vi "בדיקת מפל מתח בין הדקי הממסר תחת עומס 4.vi"(8 "error":errorcluster, 11 "Path for Log":path) -> (0 "error IO":errorcluster, 1 "בטווח כן/לא":bool, 2 "מפל מתח בין דקי הממסר תחת עומס":dbl, 3 "תוצאה זמנית":dbl)   [LabVIEW 2014]
uses:
  M9700 Driver/85/vi.lib/M9700 Modbus.llb/CTL Register Address.ctl
  M9700 Driver/86/vi.lib/M9700 Modbus.llb/CTL CMD Register.ctl
  <vilib>/DAQmx/create/channels.llb/DAQmx Create Channel (DO-Digital Output).vi
  <vilib>/DAQmx/write.llb/DAQmx Write (Digital Bool 1Line 1Point).vi
panel:
  out "progress":dbl(slide) min=0.0 max=10.0 scale=0.0..10.0
  in  "stop":bool
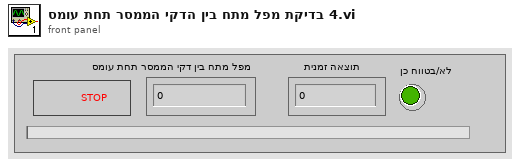
[diagram p1: front panel]
types:
  T1 = enum32{"Invalid", "Standard", "Closed", "Hidden", "Minimized", "Maximized"}
  T2 = typedef "CTL CMD Register.ctl" = u8
  T3 = typedef "CTL Register Address.ctl" = u16
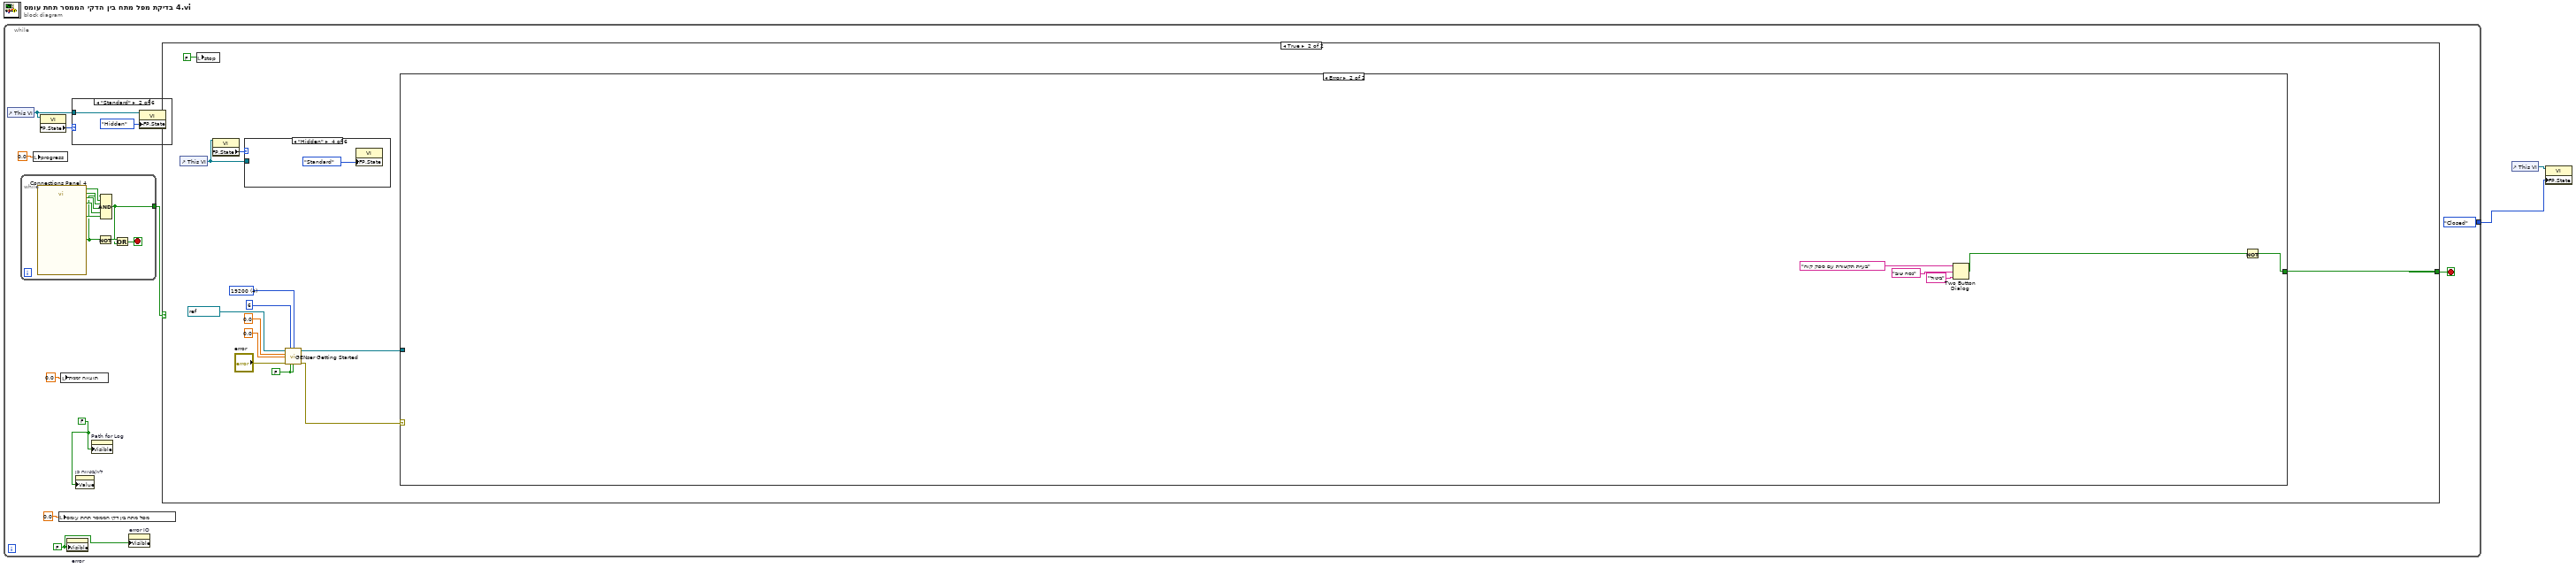
[diagram p0: block diagram]
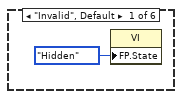
[diagram p2: hidden frame]
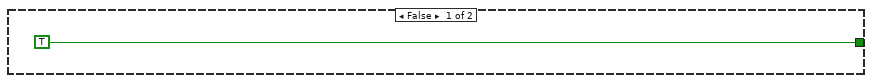
[diagram p7: hidden frame]
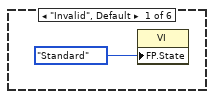
[diagram p8: hidden frame]
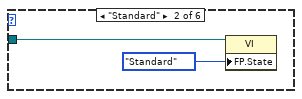
[diagram p9: hidden frame]
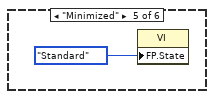
[diagram p11: hidden frame]
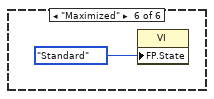
[diagram p12: hidden frame]
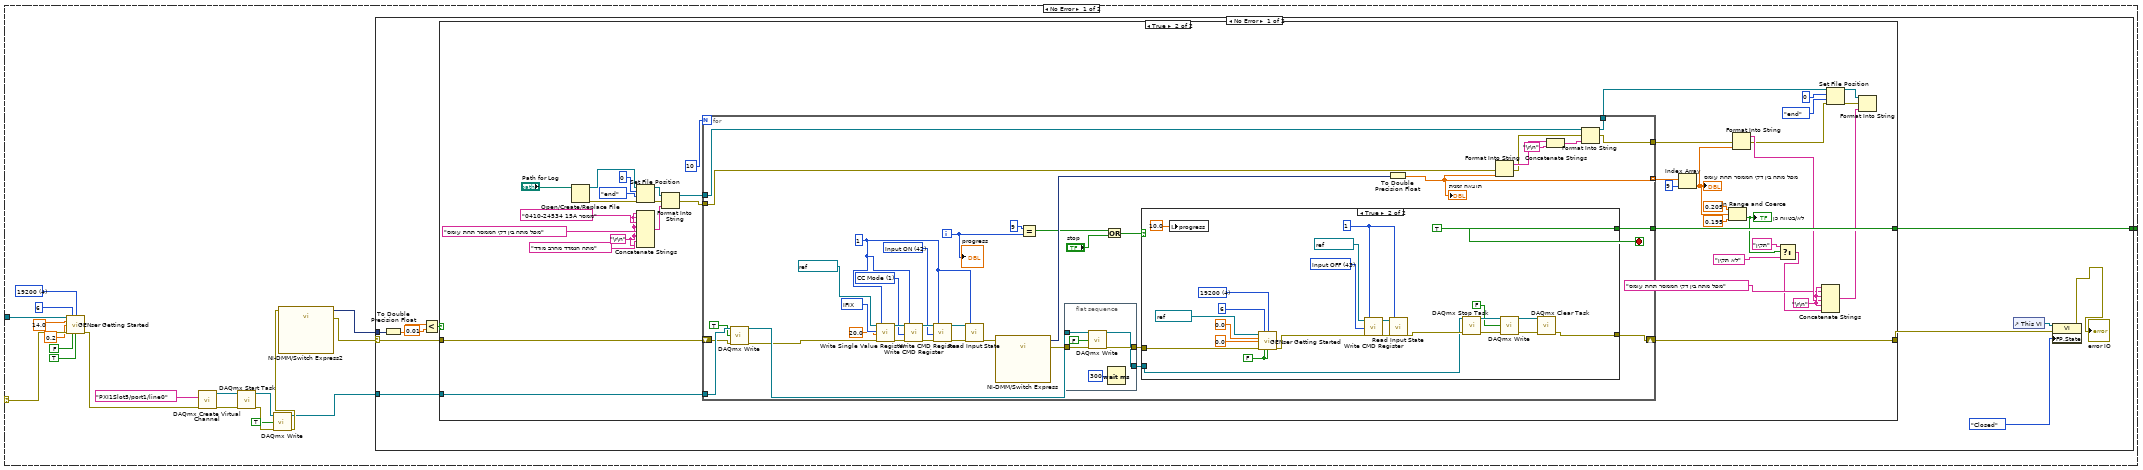
[diagram p13: hidden frame]
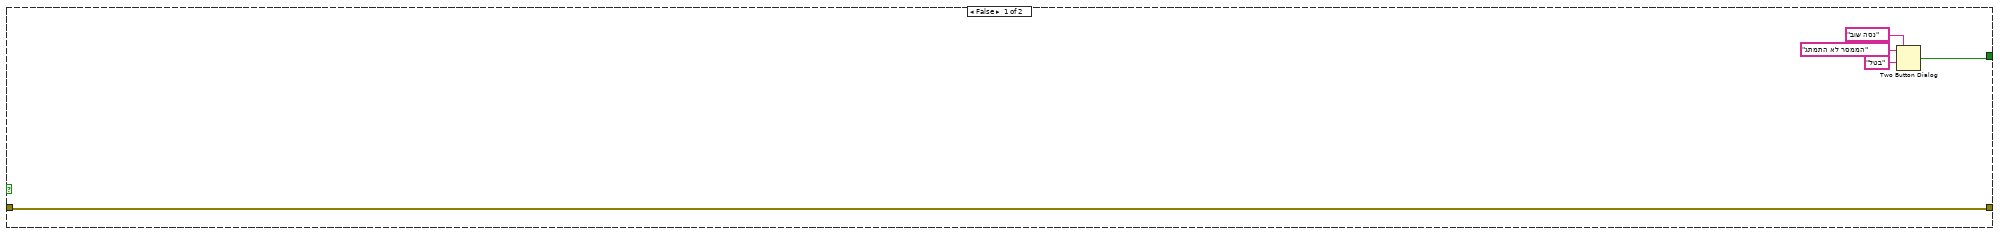
[diagram p14: hidden frame]
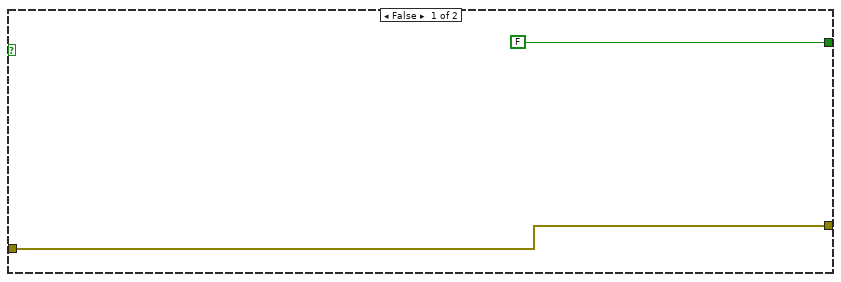
[diagram p15: hidden frame]
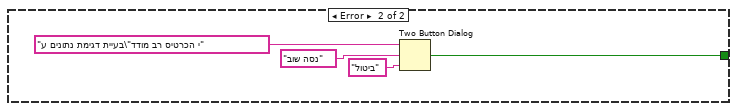
[diagram p16: hidden frame]
diagram:
  n1 = while {
    tunnel: [T1."Closed" ("Front Panel Window:State")] -> w1
    stop <- w4 stop-if-true
    w5 = FALSE ("Visible")
    w8 = FALSE ("Visible")
    n2 = control-ref of="This VI"() -> (w7:refnum<vi>)
    n3 = while {
      tunnel: [w13] -> w12
      stop <- w16 stop-if-true
      n4 = call "Connections Panel 4.vi"() -> ("Input Name 10"=w17:bool, "Input Name 6"=w21:bool, "Input Name 7"=w20:bool, "Input Name 8"=w19:bool, "Input Name 9"=w18:bool, "OK"=w14:bool)  [unwired: 13 in, 1 out]
      n5 = Not(x=w14) -> (.not. x?=w15:bool)
      n6 = Compound Arithmetic op=AND(w14, w21, w20, w19, w18, w17) -> (w13:bool)
      n7 = Or(x=w15, y=w13) -> (x .or. y?=w16:bool)
    }
    n8 = local write "progress"(0.0 ("progress")) -> ()
    n9 = property class="VI"(reference=w7) -> ("FP.State"=w6:T1)  [unwired: 1 in, 2 out]
    n10 = local write "מפל מתח בין דקי הממסר תחת עומס"(0.0 ("מפל מתח בין דקי הממסר תחת עומס")) -> ()
    n11 = local write "תוצאה זמנית"(0.0 ("תוצאה זמנית")) -> ()
    n12 = property on="error" class="Clust (strict)"("Visible"=w8) -> ()  [unwired: 2 in, 2 out]
    n13 = case shown="\"Standard\"" w6 {
      tunnel: w7 -> [_ w23 _ _ _ _]
      frame "Invalid", Default {
        n14 = property class="VI"("FP.State"=T1."Hidden" ("Front Panel Window:State")) -> ()  [unwired: 2 in, 2 out]
      }
      frame "Standard" {
        n15 = property class="VI"(reference=w23, "FP.State"=T1."Hidden" ("Front Panel Window:State")) -> ()  [unwired: 1 in, 2 out]
      }
      frame "Closed" {
      }
      frame "Hidden" {
      }
      frame "Minimized" {
      }
      frame "Maximized" {
      }
    }
    n16 = property on="בטווח כן/לא" class="Bool (strict)"("Value"=w5) -> ()  [unwired: 2 in, 2 out]
    n17 = property on="Path for Log" class="Path"("Visible"=w5) -> ()  [unwired: 2 in, 2 out]
    n18 = property on="error IO" class="Clust (strict)"("Visible"=w8) -> ()  [unwired: 2 in, 2 out]
    n19 = case shown="True" w12 {
      tunnel: [TRUE w26] -> w4
      frame False {
      }
      frame True {
        w31 = FALSE ("Output On (T)")
        w35 = u16 4 items=["1200", "2400", "4800", "9600", "19200"] ("BAUD")
        n20 = control-ref of="This VI"() -> (w28:refnum<vi>)
        n21 = local write "stop"(FALSE ("stop")) -> ()
        n22 = property class="VI"(reference=w28) -> ("FP.State"=w29:T1)  [unwired: 1 in, 2 out]
        n23 = case shown="\"Hidden\"" w29 {
          tunnel: w28 -> [_ w40 _ _ _ _]
          frame "Invalid", Default {
            n24 = property class="VI"("FP.State"=T1."Standard" ("Front Panel Window:State")) -> ()  [unwired: 2 in, 2 out]
          }
          frame "Standard" {
            n25 = property class="VI"(reference=w40, "FP.State"=T1."Standard" ("Front Panel Window:State")) -> ()  [unwired: 1 in, 2 out]
          }
          frame "Closed" {
          }
          frame "Hidden" {
            n26 = property class="VI"("FP.State"=T1."Standard" ("Front Panel Window:State")) -> ()  [unwired: 2 in, 2 out]
          }
          frame "Minimized" {
            n27 = property class="VI"("FP.State"=T1."Standard" ("Front Panel Window:State")) -> ()  [unwired: 2 in, 2 out]
          }
          frame "Maximized" {
            n28 = property class="VI"("FP.State"=T1."Standard" ("Front Panel Window:State")) -> ()  [unwired: 2 in, 2 out]
          }
        }
        n29 = call "GENser Getting Started.vi"("VISA"=refnum<visa-resource-name> "COM6", "GEN Addr"=i16 6, "BAUD"=w35, "Voltage Limit"=0.0, "Current Limit"=0.0, "error"="error", "Reset (T)"=w31, "Output On (T)"=w31) -> ("VISA out"=w37:refnum<visa-resource-name>, "error out"=w27:errorcluster)  [unwired: 4 in, 2 out]
        n30 = case shown="Error" w27 {
          selector: w27 -> [w61 _]
          tunnel: w37 -> [w64 _]
          tunnel: [w63 w193] -> w26
          frame No Error {
            w55 = u16 4 items=["1200", "2400", "4800", "9600", "19200"] ("BAUD")
            n31 = call "GENser Getting Started.vi"("VISA"=w64, "GEN Addr"=i16 6, "BAUD"=w55, "Voltage Limit"=14.0, "Current Limit"=0.2, "error"=w61, "Reset (T)"=FALSE, "Output On (T)"=TRUE) -> ("error out"=w47:errorcluster)  [unwired: 4 in, 3 out]
            n32 = call-poly <vilib>:"DAQmx Create Virtual Channel.vi"("lines"=tag "PXI1Slot5/port1/line0", "error in"=w47) -> ("task out"=w53:refnum<k21>, "error out"=w54:errorcluster)  [unwired: 12 in]
            n33 = call <vilib>:"DAQmx Start Task.vi"("task/channels in"=w53, "error in"=w54) -> ("task out"=w46:refnum<k21>, "error out"=w49:errorcluster)  [unwired: 12 in]
            n34 = call-poly <vilib>:"DAQmx Write.vi"("task/channels in"=w46, "data"=TRUE, "error in"=w49) -> ("task out"=w45:refnum<k21>, "error out"=w50:errorcluster)  [unwired: 10 in, 1 out]
            n35 = call "NI-DMM/Switch Express2"("error in"=w50) -> ("signals out"=w62:dynamicdata, "error out"=w51:errorcluster)  [unwired: 16 in, 1 out]
            n36 = case shown="No Error" w51 {
              selector: w51 -> [w73 _]
              tunnel: [w72 w189] -> w63
              tunnel: w62 -> [w75 _]
              tunnel: w45 -> [w66 _]
              frame No Error {
                n37 = To Double Precision Float(number=w75) -> (double precision float=w71:dbl)
                n38 = Less?(x=w71, y=0.01) -> (x < y?=w74:bool)
                n39 = case shown="True" w74 {
                  tunnel: w73 -> [w80 w117]
                  tunnel: [w79 w118] -> w72
                  tunnel: [w80 w111] -> w67
                  tunnel: w66 -> [_ w112]
                  frame False {
                    n40 = Two Button Dialog(message="הממסר לא התמתג", 1:"נסה שוב" ("F button name (\"Cancel\")"), 2:"בטל" ("T button name (\"OK\")")) -> (T button?=w79:bool)
                  }
                  frame True {
                    w96 = "\r\n"
                    w99 = "\r\n"
                    n41 = Open/Create/Replace File(file path (use dialog)="Path for Log") -> (refnum out=w108:refnum<file>, error out=w107:errorcluster)  [unwired: 5 in, 1 out]
                    n42 = Set File Position(offset (in bytes) (0)=i64 0, refnum=w108, from (0:start)=enum16{"start", "end", "current"}."end", error in=w107) -> (refnum out=w103:refnum<file>, error out=w100:errorcluster)
                    n43 = Concatenate Strings(w99, w99, "0410-24534 15A ממסר", w99, "מפל מתח בין דקי הממסר תחת עומס", w99, "מתח הנמדד מהרב מודד", w99) -> (w106:string)
                    n44 = Format Into String(initial string=w103, error in=w100, w106) -> (resulting string=w97:refnum<file>, error out=w98:errorcluster)  [unwired: 1 in]
                    n45 = for {
                      N: 10 -> [_]
                      tunnel: [w140] -> w118
                      shift-right: [w138] -> w111
                      shift-left: w117 -> [w133]
                      tunnel: [w121] -> w116 mode=indexing
                      tunnel: w112 -> [w134]
                      tunnel: w98 -> [w124]
                      tunnel: w97 -> [w126]
                      tunnel: [w123] -> w90
                      tunnel: [w122] -> w81
                      i -> [w137]
                      stop <- w140 stop-if-true
                      w148 = T2 42 items=["CC Mode"=1, "CV Mode"=2, "CW Mode"=3, "CR Mode"=4, "Short Mode"=26, "Set SysPara"=41, "Input ON"=42, "Input OFF"=43] ("CMD Register Value")
                      w151 = u8 1 ("Load Address")
                      w154 = T2 1 items=["CC Mode"=1, "CV Mode"=2, "CW Mode"=3, "CR Mode"=4, "Short Mode"=26, "Set SysPara"=41, "Input ON"=42, "Input OFF"=43] ("CMD Register Value")
                      w157 = T3 2561 items=["REMOTE"=1283, "ISTATE"=1296, "CMD"=2560, "IFIX"=2561, "UFIX"=2563, "PFIX"=2565, "RFIX"=2567, "IMAX"=2612, "UMAX"=2614, "PMAX"=2616, "U"=2816, "I"=2818, "MODEL"=2822, "EDITION"=2823] ("Register Address")
                      n46 = call-poly <vilib>:"DAQmx Write.vi"("task/channels in"=w134, "data"=TRUE, "error in"=w133) -> ("task out"=w132:refnum<k21>, "error out"=w120:errorcluster)  [unwired: 10 in, 1 out]
                      n47 = call "Write Single Value Register.vi"("VISA resource name"=refnum<visa-resource-name> "COM13", "Starting Address(HEX)"=w157, "Register Single Value"=sgl 20.0, "error in"=w120, "Load Address"=w151) -> ("VISA resource name out"=w156:refnum<visa-resource-name>, "error out"=w155:errorcluster)  [unwired: 13 out]
                      n48 = call "Write CMD Register.vi"("VISA resource name"=w156, "CMD Value"=w154, "error in"=w155, "Load Address"=w151) -> ("VISA resource name out"=w152:refnum<visa-resource-name>, "error out"=w149:errorcluster)  [unwired: 14 out]
                      n49 = call "Write CMD Register.vi"("VISA resource name"=w152, "CMD Value"=w148, "error in"=w149, "Load Address"=w151) -> ("VISA resource name out"=w150:refnum<visa-resource-name>, "error out"=w147:errorcluster)  [unwired: 14 out]
                      n50 = call "Read Input State.vi"("VISA resource name"=w150, "error in"=w147, "Load Address"=w151) -> ("error out"=w146:errorcluster)  [unwired: 16 out]
                      n51 = call "NI-DMM/Switch Express"("error in"=w146) -> ("signals out"=w145:dynamicdata, "error out"=w135:errorcluster)  [unwired: 16 in, 1 out]
                      n52 = Equal?(x=9, y=w137) -> (x = y?=w142:bool)
                      n53 = flat-sequence {
                        tunnel: [w163] -> w136
                        tunnel: w135 -> [w162]
                        tunnel: w132 -> [w160]
                        tunnel: [w159] -> w130
                        frame #0 {
                          n54 = call-poly <vilib>:"DAQmx Write.vi"("task/channels in"=w160, "data"=FALSE, "error in"=w162) -> ("task out"=w159:refnum<k21>, "error out"=w163:errorcluster)  [unwired: 10 in, 1 out]
                          n55 = Wait (ms)(milliseconds to wait=u32 300) -> ()  [unwired: 1 out]
                        }
                      }
                      n56 = Or(x=w142, y="stop") -> (x .or. y?=w143:bool)
                      n57 = case shown="True" w143 {
                        tunnel: [FALSE TRUE] -> w140
                        tunnel: w136 -> [w164 w182]
                        tunnel: [w164 w168] -> w138
                        tunnel: w130 -> [_ w167]
                        frame False {
                        }
                        frame True {
                          w176 = u8 1 ("Load Address")
                          w179 = T2 43 items=["CC Mode"=1, "CV Mode"=2, "CW Mode"=3, "CR Mode"=4, "Short Mode"=26, "Set SysPara"=41, "Input ON"=42, "Input OFF"=43] ("CMD Register Value")
                          w181 = FALSE ("Reset (T)")
                          w184 = u16 4 items=["1200", "2400", "4800", "9600", "19200"] ("BAUD")
                          n58 = local write "progress"(10.0 ("progress")) -> ()
                          n59 = call "GENser Getting Started.vi"("VISA"=refnum<visa-resource-name> "COM6", "GEN Addr"=i16 6, "BAUD"=w184, "Voltage Limit"=0.0, "Current Limit"=0.0, "error"=w182, "Reset (T)"=w181, "Output On (T)"=w181) -> ("error out"=w166:errorcluster)  [unwired: 4 in, 3 out]
                          n60 = call "Write CMD Register.vi"("VISA resource name"=refnum<visa-resource-name> "COM13", "CMD Value"=w179, "error in"=w166, "Load Address"=w176) -> ("VISA resource name out"=w177:refnum<visa-resource-name>, "error out"=w180:errorcluster)  [unwired: 14 out]
                          n61 = call "Read Input State.vi"("VISA resource name"=w177, "error in"=w180, "Load Address"=w176) -> ("error out"=w169:errorcluster)  [unwired: 16 out]
                          n62 = call <vilib>:"DAQmx Stop Task.vi"("task/channels in"=w167, "error in"=w169) -> ("task out"=w174:refnum<k21>, "error out"=w172:errorcluster)  [unwired: 12 in]
                          n63 = call-poly <vilib>:"DAQmx Write.vi"("task/channels in"=w174, "data"=FALSE, "error in"=w172) -> ("task out"=w171:refnum<k21>, "error out"=w170:errorcluster)  [unwired: 10 in, 1 out]
                          n64 = call <vilib>:"DAQmx Clear Task.vi"("task in"=w171, "error in"=w170) -> ("error out"=w168:errorcluster)  [unwired: 13 in]
                        }
                      }
                      n65 = To Double Precision Float(number=w145) -> (double precision float=w121:dbl)
                      "תוצאה זמנית" <- w121
                      n66 = Format Into String(error in=w124, w121) -> (resulting string=w128:string, error out=w125:errorcluster)  [unwired: 2 in]
                      n67 = Concatenate Strings(w128, "\r\n") -> (w127:string)
                      n68 = Format Into String(initial string=w126, error in=w125, w127) -> (resulting string=w123:refnum<file>, error out=w122:errorcluster)  [unwired: 1 in]
                      "progress" <- w137
                    }
                    n69 = Index Array(array=w116, index=9) -> (element=w89:dbl)
                    "מפל מתח בין דקי הממסר תחת עומס" <- w89
                    n70 = In Range and Coerce(upper limit=0.205, x=w89, lower limit=0.195) -> (In Range?=w84:bool)  [unwired: 1 out]
                    "בטווח כן/לא" <- w84
                    n71 = Format Into String(error in=w81, w89) -> (resulting string=w88:string, error out=w82:errorcluster)  [unwired: 2 in]
                    n72 = Select(t="תקין", s=w84, f="לא תקין") -> (s? t:f=w83:string)
                    n73 = Concatenate Strings(w96, "מפל מתח בין דקי הממסר תחת עומס" ("string"), w96, w88, w96, w83) -> (w91:string)
                    n74 = Set File Position(offset (in bytes) (0)=i64 0, refnum=w90, from (0:start)=enum16{"start", "end", "current"}."end", error in=w82) -> (refnum out=w93:refnum<file>, error out=w92:errorcluster)
                    n75 = Format Into String(initial string=w93, error in=w92, w91) -> ()  [unwired: 1 in, 2 out]
                  }
                }
                n76 = control-ref of="This VI"() -> (w69:refnum<vi>)
                n77 = property class="VI"(reference=w69, error in=w67, "FP.State"=T1."Closed" ("Front Panel Window:State")) -> (error out=→"error IO":errorcluster)  [unwired: 1 out]
              }
              frame Error {
                n78 = Two Button Dialog(message="בעיית דגימת נתונים ע\"י הכרטיס רב מודד", 1:"ביטול" ("F button name (\"Cancel\")"), 2:"נסה שוב" ("T button name (\"OK\")")) -> (T button?=w189:bool)
              }
            }
          }
          frame Error {
            n79 = Two Button Dialog(message="בעיית תקשורת עם ספק קוח", 1:"ביטול" ("F button name (\"Cancel\")"), 2:"נסה שוב" ("T button name (\"OK\")")) -> (T button?=w194:bool)
            n80 = Not(x=w194) -> (.not. x?=w193:bool)
          }
        }
      }
    }
  }
  n81 = control-ref of="This VI"() -> (w2:refnum<vi>)
  n82 = property class="VI"(reference=w2, "FP.State"=w1) -> ()  [unwired: 1 in, 2 out]
